vi "NVH_TEST.vi"(10 "振动2NHV-FFT":refnum<vi>, 11 "振动1NVH-FFT":refnum<vi>) -> ()   [LabVIEW 2020]
uses:
  Global_Variable/Global.vi
panel:
  out "error out":errorcluster caption="错误输出"
  in  "error in":errorcluster caption="错误输入"
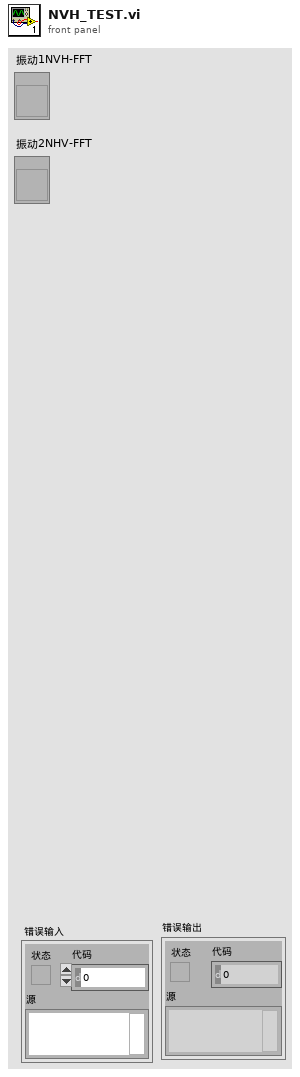
[diagram p1: front panel]
types:
  T1 = typedef "svc_Spectrum Info.ctl" = cluster{"channel name":string, "description":string, "x-axis units":T2, "spectral info":cluster{"spectrum type":T3, "linear/dB":enum16{"linear", "dB"}, "window":u16, "window size":i32, "FFT size":i32}, "engineering units":T4, "custom label":string, "dB reference [EU]":dbl, "peak units":enum16{"rms", "peak", "peak-peak"}, "weighting filter":T5, "spectral density?":bool, "unit label":string, "spectrum skewed?":bool, "complimentary spectrum units":T6}
  T2 = typedef "svc_X-Axis Units.ctl" = u16
  T3 = typedef "svc_Spectrum Type.ctl" = enum16{"FFT Spectrum [complex]", "Amplitude [Magnitude]", "Power [Magnitude^2]", "Cross Spectrum [complex]", "Frequency Response [Complex]"}
  T4 = typedef "svc_Engineering Units Text Ring.ctl" = u16
  T5 = typedef "svc_Weighting Filter Text Ring.ctl" = u16
  T6 = typedef "svc_Complimentary Spectrum Units.ctl" = enum16{"none", "radians", "degrees", "cycles", "imaginary"}
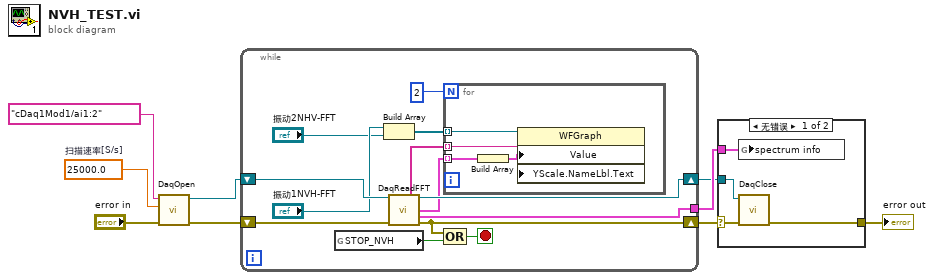
[diagram p0: block diagram]
diagram:
  w1 = 25000.0  # 扫描速率[S/s]
  n1 = call "DaqOpen.vi"("error in"="error in", "扫描速率[S/s]"=w1, "通道输入"=tag "cDaq1Mod1/ai1:2" ("DAQmx物理通道")) -> ("error out"=w9:errorcluster, "task out"=w3:refnum<k21>)  [unwired: 7 in]
  n2 = while {
    shift-right: [w21] -> w4
    shift-left: w3 -> [w22]
    shift-right: [w20] -> w5
    shift-left: w9 -> [w17]
    tunnel: [w18] -> w7
    stop <- w19 stop-if-true
    n3 = global read "Global.vi" "STOP_NVH"() -> (w16:bool)
    n4 = Build Array("振动1NVH-FFT", "振动2NHV-FFT") -> (w13:refnum<vi>[])
    n5 = call "DaqReadFFT.vi"("任务输入"=w22, "error in"=w17) -> ("unit labels"=w11:string[], "task out 2"=w21:refnum<k21>, "power spectra [dB EU]"=w12:cluster{"f0":dbl, "df":dbl, "magnitude":dbl[]}[], "spectrum info"=w18:T1[], "error out"=w20:errorcluster)  [unwired: 8 in, 1 out]
    n6 = for {
      N: 2 -> [_]
      tunnel: w13 -> [w26] mode=indexing
      tunnel: w12 -> [w25] mode=indexing
      tunnel: w11 -> [w24] mode=indexing
      n7 = Build Array(w25) -> (w23:cluster{"f0":dbl, "df":dbl, "magnitude":dbl[]}[])
      n8 = property class="WFGraph"(reference=w26, "Value"=w23, "YScale.NameLbl.Text"=w24) -> ()  [unwired: 1 in, 2 out]
    }
    n9 = Compound Arithmetic op=OR ("复合运算")(w20, w16) -> (w19:bool)
  }
  n10 = case shown="无错误" w5 {
    selector: w5 -> [w29 w31]
    tunnel: w4 -> [w30 _]
    tunnel: [w28 w31] -> w6
    tunnel: w7 -> [w27 _]
    frame No Error {
      n11 = global write "Global.vi" "spectrum info"(w27) -> ()
      n12 = call "DaqClose.vi"("error in"=w29, "task in"=w30) -> ("error out"=w28:errorcluster)  [unwired: 9 in]
    }
    frame Error {
    }
  }
  "error out" <- w6
